vi "host-C-Experimental.vi"() -> (0 "K(Indicator)":fxp<+/-,64,32>=1.52587890625e-05, 1 "degree":dbl=0.1952712924057206, 2 "Nominal Freq":fxp<+/-,64,32>=0.494873046875)   [LabVIEW 2012]
uses:
  <vilib>/addons/control/pid/pid.llb/PID (DBL).vi
  <vilib>/Utility/file.llb/Write To Spreadsheet File (DBL).vi
  <vilib>/Utility/file.llb/Write To Spreadsheet File (I64).vi
  <vilib>/FPGAPlugInAG/PCI-7831R/niLvFpga_Open_PCI-7831R.vi
  <vilib>/rvi/interface/common/dynamic/niFpgaDynamicAddResources.vi
  <vilib>/Utility/error.llb/Error Cluster From Error Code.vi
  <vilib>/rvi/errors/niLvFpgaAdjustHostInterfaceError.vi
  <vilib>/FPGAPlugInAG/Dynamic/niLvFpga_Abort_Dynamic.vi
  <vilib>/FPGAPlugInAG/Dynamic/niLvFpga_Close_Dynamic.vi
  <vilib>/FPGAPlugInAG/PCI-7831R/niLvFpga_Abort_PCI-7831R.vi
  <vilib>/FPGAPlugInAG/PCI-7831R/niLvFpga_Close_PCI-7831R.vi
  <vilib>/FPGAPlugInAG/PCI-7831R/niLvFpga_Run_PCI-7831R.vi
  <vilib>/rvi/interface/nirviOpenFPGA/nirviOpenFPGA.xnode
  SB130-XPS/Documents/FPGA-project-apporach-retraction/FPGA Bitfiles/Apporach-Retract_FPGATarget_LIAFPGA3a-PDTest_MjY0boR9VLg.lvbitx
  Documents/Pramith_Computer/FPGA PLL/LIA_FPGA3a-PD Test-3.vi
  <vilib>/rvi/interface/nirviReadWriteControl/nirviReadWriteControl.xnode
  <vilib>/rvi/interface/nirviMethod/nirviMethod.xnode
  <vilib>/rvi/interface/nirviCloseFPGA/nirviCloseFPGA.xnode
  <vilib>/rvi/errors/niLvFpgaMergeErrorWithErrorCode.vi
  NiFpgaLv.dll
  <vilib>/FPGAPlugInAG/Dynamic/niLvFpga_StartFifo_Dynamic.vi
  <vilib>/FPGAPlugInAG/Dynamic/niLvFpga_StopFifo_Dynamic.vi
  <vilib>/rvi/interface/Simulation/niFpgaSimulationCallBeginRW.vi
  <vilib>/FPGAPlugInAG/Dynamic/niLvFpga_ReadFifo_Dynamic.vi
  <vilib>/addons/control/pid/NI_PID_pid.lvlib
panel:
  out "Output":dbl
  in  "Proportional Constant":dbl
  in  "Reinitialize":bool
  out "Numeric 2":dbl
  out "Corrected Frequency 2":dbl
  out "P+I Error 2":dbl
  in  "VCO Constant 2":dbl=0.010000000000000009
  out "Numeric 3":fxp<+/-,64,32>
  out "Sig Gen Frequency":dbl
  out "Corrected Frequency":fxp<+/-,64,32>
  out "Angular Frequency":fxp<+/-,64,32>
  out "Z Error":fxp<+/-,64,32>
  in  "VCO Constant":fxp<+/-,64,10>=0.010000000000000009
  in  "Proportional Gain":fxp<+/-,64,32>=0.0009999999310821295
  in  "Integral Gain":fxp<+/-,64,32>=0.0009999999310821295
  out "P+I Error":fxp<+/-,64,32>
  out "PID Input Error":dbl
  out "Phase (Degree) Shift":fxp<+/-,64,32>
  out "Numeric":fxp<+/-,64,32>
  out "For Proportional":fxp<+/-,64,32>
  out "Case Number":i16
  in  "Signal Generator":bool
  in  "PID":bool
  in  "Voltage (V)":dbl=0.03
  in  "Frequency":dbl=32767.0
  out "Waveform Chart 2":i32[](graph)
  out "Waveform Chart":i32[](graph)
  in  "Number of Elements":i32
  in  "Path 5":path
  in  "name-file 11":string="approach-15a"
  out "String 11":string
  in  "Path 7":path
  in  "name-file 9":string="approach-15a"
  out "String 9":string
  in  "Path 4":path
  in  "name-file 4":string="approach-15a"
  out "String 4":string
  in  "Path 3":path
  in  "name-file 3":string="approach-15a"
  out "String 3":string
  in  "Path 2":path
  in  "name-file 2":string="approach-15a"
  out "String 2":string
  in  "Data Collector":bool
  out "String":string
  in  "name-file":string="approach-15a"
  in  "Path":path
  out "Standardized nominal freq":dbl
  in  "Delta Nominal Frequency":dbl
  out "Ref":i32
  out "Sig":i32
  out "Sin":dbl(graph)
  out "Phase":dbl
  out "Ze Output":dbl=2.3841857910156248e-12
  out "The Decs":dbl=7.8125e-09
  out "LSB Weight":dbl=0.00030517578125
  in  "K":fxp<+,16,0>=6.103515625e-05
  in  "nominal freq 2":fxp<+,16,0>=0.494873046875
  out "x*y":dbl=0.015
  in  "stop 2":bool
  out "3rd stages":i32=1
  out "3rd decimation":i32=977
  out "1st decimation":i32=1
  out "2nd decimation":i32=128
  in  "Time Constant [s]":dbl=2.5 min=0.0 step=0.0001 format="%.2f"
  in  "Filter Rolloff":enum16{"20 dB", "40 dB", "60 dB", "80 dB"}(ring)
  out "Actual Sampling Frequency":dbl=200000.0
  in  "input range of 9205":dbl=10.0
  in  "Sampling Frequency":dbl=200000.0 min=1000.0 max=250000.0
  in  "stop":bool
  out "r":dbl(graph)=0.5098420210496609
  out "y":dbl=0.0017376029872894286
  out "x":dbl=0.5098390600609779
  out "f":dbl(graph)=31000.332441180944
  in  "dec2":i16=1
  in  "nominal freq":dbl=30000.0 min=500.0 max=125000.0
  in  "dec1":i16=1000
  in  "stages":i8=1 min=1 max=2
  in  "decimation":i16=1000
  # "Sampling Frequency"
  # "CIC First Decimation"
  # "MA Stages"
  # "CIC Second Decimation"
  # "PLL Nominal Frequency"
  # "MA Decimation"
  # "PLL Frequency Output"
  # "LIA Output"
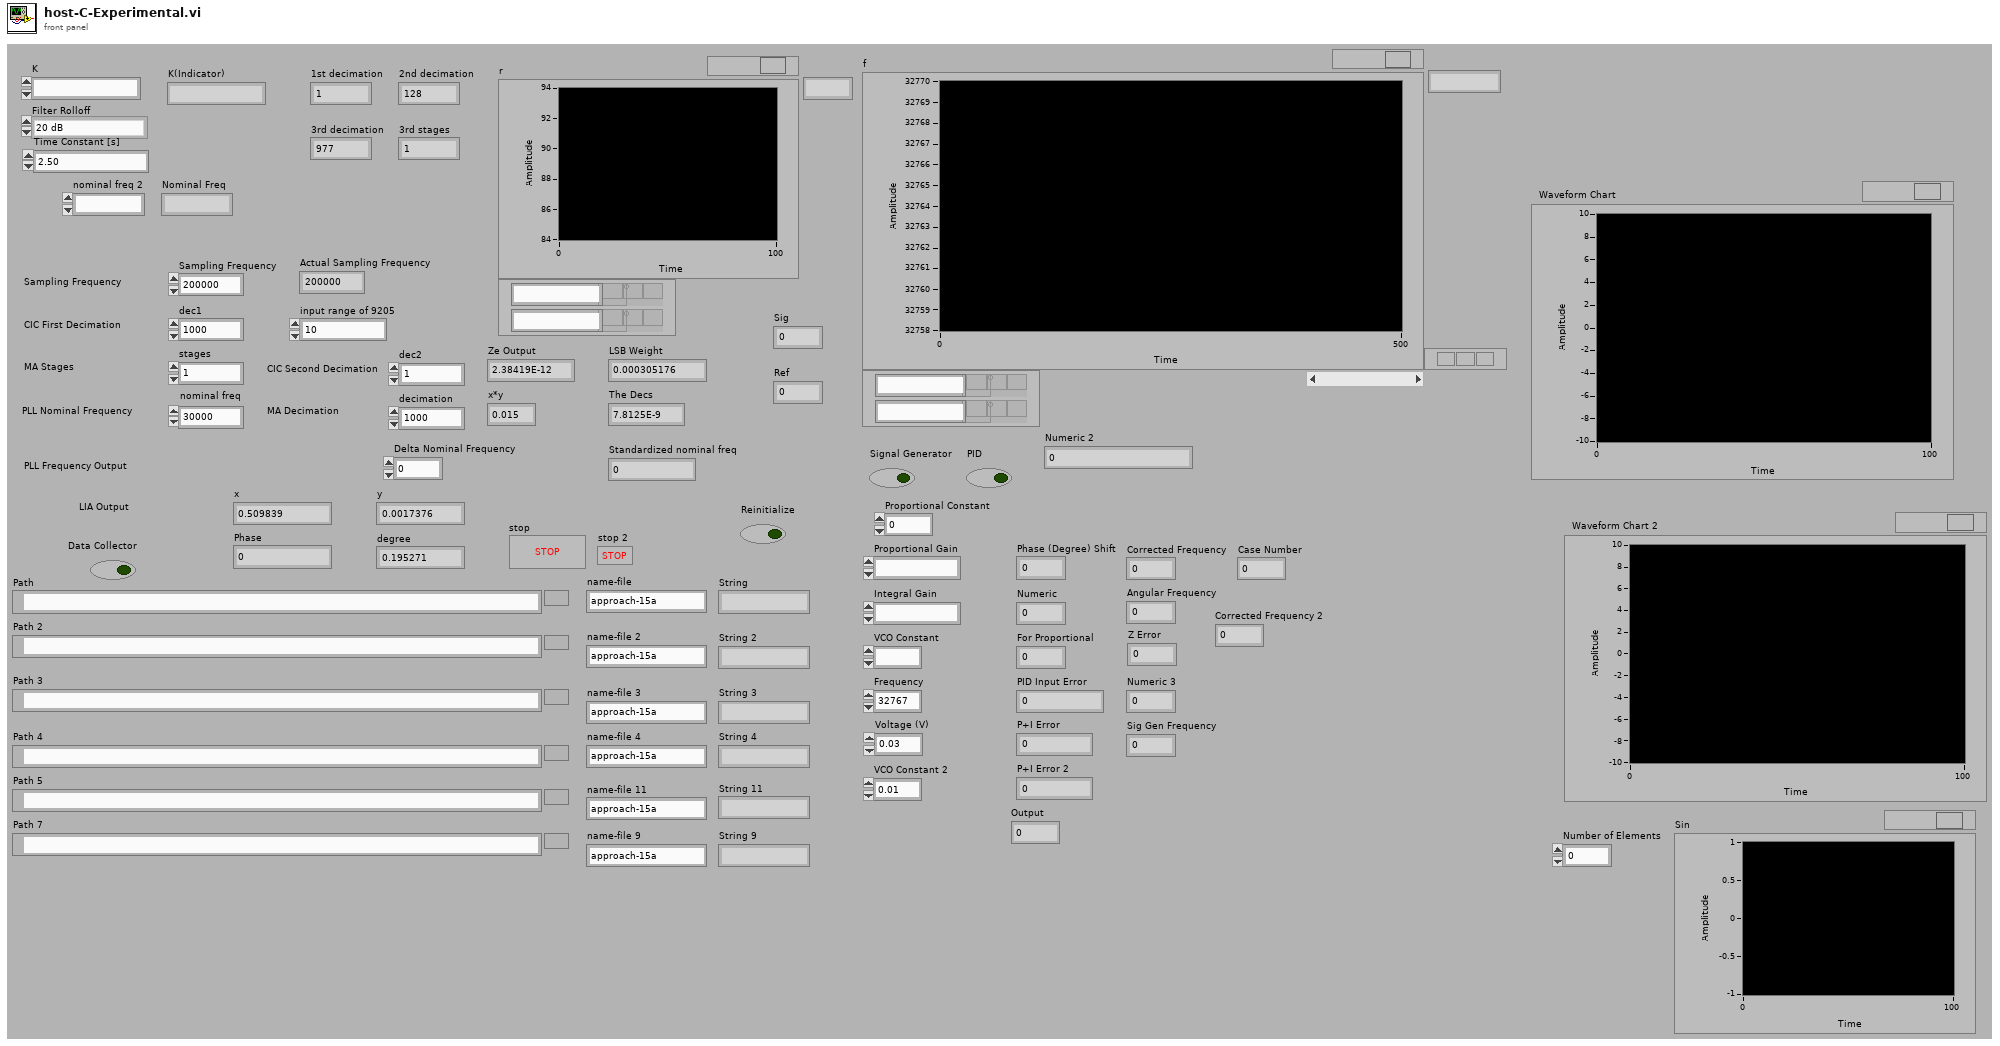
[diagram p1: front panel]
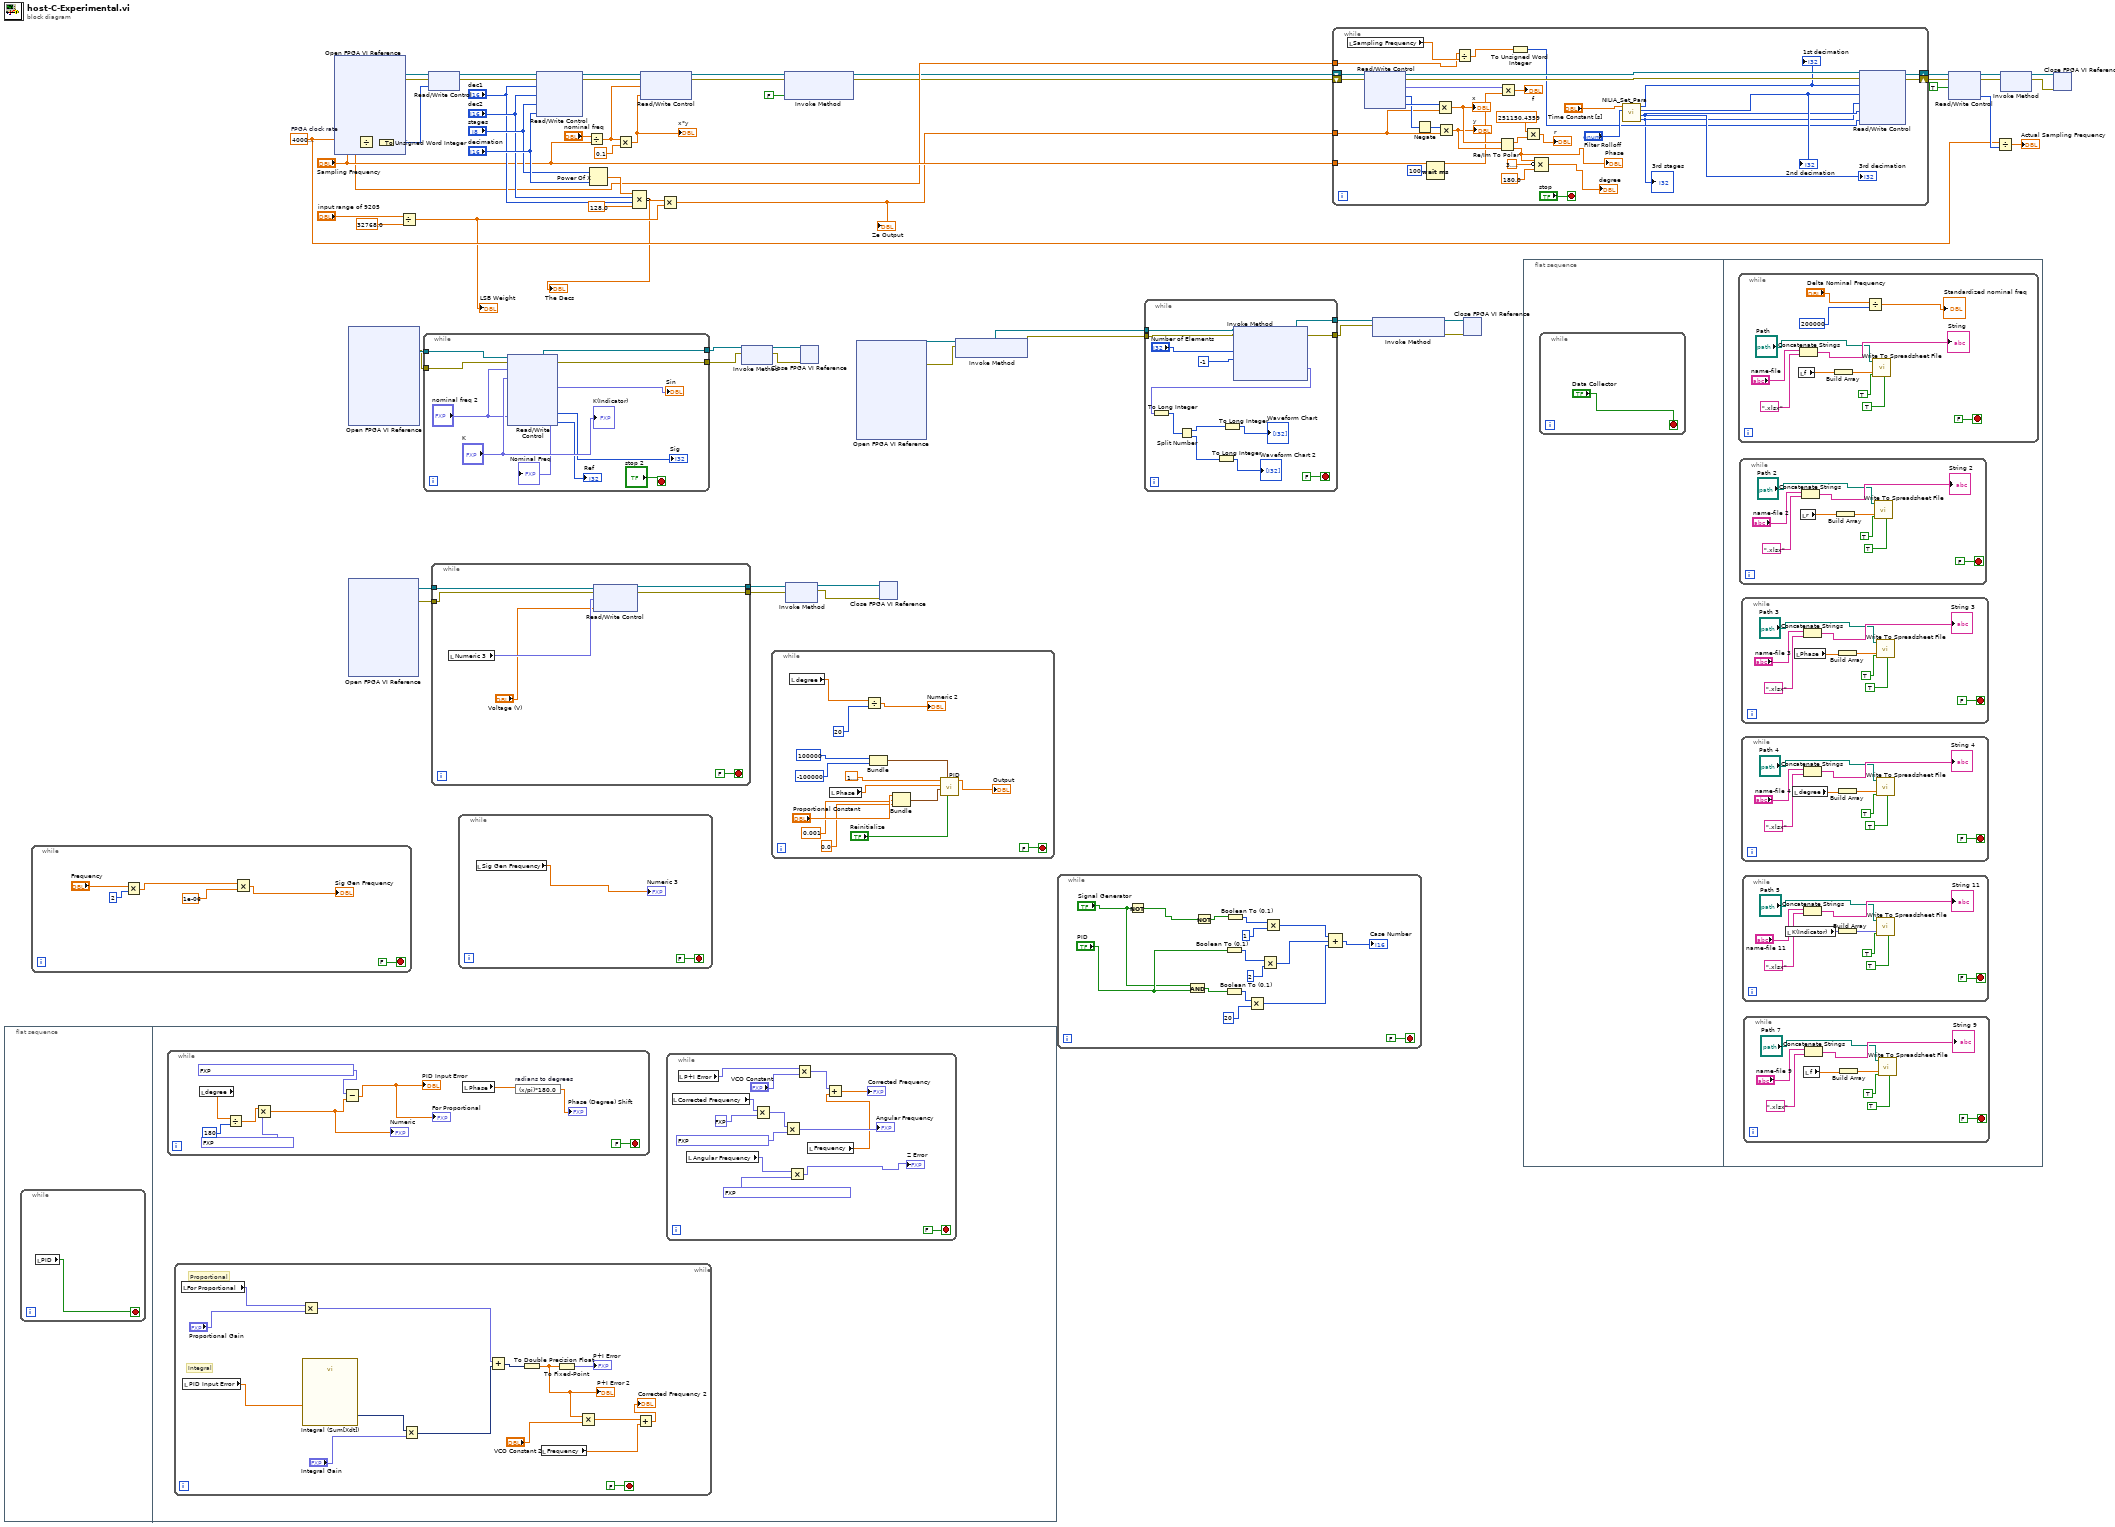
[diagram p0: block diagram]
diagram:
  w29 = 40000000.0  # FPGA clock rate
  n1 = flat-sequence {
    frame #0 {
      n2 = while {
        stop <- w60 stop-if-true
        n3 = local read "PID"() -> (w60:bool)
      }
    }
    frame #1 {
      n4 = while {
        stop <- FALSE stop-if-true
        n5 = local read "degree"() -> (w90:dbl)
        n6 = Divide(x=w90, y=i16 180) -> (x/y=w98:dbl)
        n7 = Multiply(x=w98, y=fxp<+,30,2> 3.1415926814079285) -> (x*y=w97:dbl)
        "Numeric" <- w97
        n8 = Subtract(x=fxp<+,50,1> 1.5707963199999995, y=w97) -> (x-y=→"PID Input Error" →"For Proportional":dbl)
        n9 = local read "Phase"() -> (w92:dbl)
        n10 = expression code="(x/pi)*180.0" "radians to degrees"(w92) -> (→"Phase (Degree) Shift":dbl)
      }
      n11 = while {
        stop <- FALSE stop-if-true
        # "Integral"
        # "Proportional"
        n12 = local read "For Proportional"() -> (w89:fxp<+/-,64,32>)
        n13 = local read "PID Input Error"() -> (w87:dbl)
        n14 = Multiply(x=w89, y="Proportional Gain") -> (x*y=w84:fxp<+/-,64,64>)
        n15 = call "Integral (Sum[Xdt])"("Signals"=w87) -> ("Result"=w86:dynamicdata)  [unwired: 5 in, 1 out]
        n16 = Multiply(x=w86, y="Integral Gain") -> (x*y=w83:dynamicdata)
        n17 = Add(x=w84, y=w83) -> (x+y=w82:dynamicdata)
        n18 = To Double Precision Float(number=w82) -> (double precision float=w79:dbl)
        "P+I Error 2" <- w79
        n19 = local read "Frequency"() -> (w76:dbl)
        n20 = To Fixed-Point(number=w79) -> (fixed-point=→"P+I Error":fxp<+/-,32,16>)  [unwired: 1 in]
        n21 = Multiply(x=w79, y="VCO Constant 2") -> (x*y=w77:dbl)
        n22 = Add(x=w77, y=w76) -> (x+y=→"Corrected Frequency 2":dbl)
      }
      n23 = while {
        stop <- FALSE stop-if-true
        n24 = local read "Corrected Frequency"() -> (w67:fxp<+/-,64,32>)
        n25 = local read "P+I Error"() -> (w63:fxp<+/-,64,32>)
        n26 = local read "Angular Frequency"() -> (w72:fxp<+/-,64,32>)
        n27 = Multiply(x=w67, y=fxp<+,1,2> 2.0) -> (x*y=w70:fxp<+/-,64,33>)
        n28 = Multiply(x=w70, y=fxp<+,30,2> 3.1415926814079285) -> (x*y=→"Angular Frequency":fxp<+/-,64,35>)
        n29 = Multiply(x=w72, y=fxp<+,46,7> 1.0000003385357559e-06) -> (x*y=→"Z Error":fxp<+/-,64,39>)
        n30 = Multiply(x=w63, y="VCO Constant") -> (x*y=w65:fxp<+/-,64,42>)
        n31 = local read "Frequency"() -> (w62:dbl)
        n32 = Add(x=w65, y=w62) -> (x+y=→"Corrected Frequency":dbl)
      }
    }
  }
  n33 = while {
    stop <- FALSE stop-if-true
    n34 = Multiply(x="Frequency", y=2) -> (x*y=w105:dbl)
    n35 = Multiply(x=w105, y=1e-06) -> (x*y=→"Sig Gen Frequency":dbl)
  }
  n36 = xnode "Open FPGA VI Reference"() -> ("FPGA VI Reference Out"=w35:refnum<k20>, "error out"=w34:errorcluster)  [unwired: 2 in]
  n37 = xnode ("Open FPGA VI Reference")() -> ("FPGA VI Reference Out"=w6:refnum<k20>, "error out"=w5:errorcluster)  [unwired: 2 in]
  n38 = xnode "Open FPGA VI Reference"() -> ("FPGA VI Reference Out"=w28:refnum<k20>, "error out"=w27:errorcluster)  [unwired: 2 in]
  n39 = Divide(x=w29, y="Sampling Frequency") -> (x/y=w41:dbl)
  n40 = To Unsigned Word Integer(number=w41) -> (unsigned 16bit integer=w40:u16)
  n41 = Divide(x="input range of 9205", y=32768.0) -> (x/y=w21:dbl)
  "LSB Weight" <- w21
  n42 = while {
    tunnel: w28 -> [w114]
    tunnel: w27 -> [w113]
    tunnel: [w112] -> w26
    tunnel: [w111] -> w25
    stop <- "stop 2" stop-if-true
    n43 = xnode "Read/Write Control"("FPGA VI Reference In"=w114, "error in"=w113, "nominal freq"="nominal freq 2", "K"="K") -> ("FPGA VI Reference Out"=w112:refnum<k20>, "error out"=w111:errorcluster, "Sin"=→"Sin":fxp<+/-,14,2>, "sig"=→"Sig":i16, "ref"=→"Ref":i16)  [unwired: 2 out]
    "K(Indicator)" <- "K"
    "Nominal Freq" <- "nominal freq 2"
  }
  n44 = xnode "Read/Write Control"("FPGA VI Reference In"=w35, "error in"=w34, "Period"=w40) -> ("FPGA VI Reference Out"=w43:refnum<k20>, "error out"=w42:errorcluster)
  n45 = while {
    tunnel: w6 -> [w121]
    tunnel: w5 -> [w120]
    tunnel: [w119] -> w4
    tunnel: [w118] -> w3
    stop <- FALSE stop-if-true
    n46 = local read "Numeric 3"() -> (w117:fxp<+/-,64,32>)
    n47 = xnode "Read/Write Control"("FPGA VI Reference In"=w121, "error in"=w120, "Z"=w117, "Voltage (V)"="Voltage (V)") -> ("FPGA VI Reference Out"=w119:refnum<k20>, "error out"=w118:errorcluster)
  }
  n48 = while {
    stop <- FALSE stop-if-true
    n49 = local read "Sig Gen Frequency"() -> (→"Numeric 3":dbl)
  }
  n50 = xnode "Read/Write Control"("FPGA VI Reference In"=w43, "error in"=w42, "dec1"="dec1", "dec2"="dec2", "stages"="stages", "decimation"="decimation") -> ("FPGA VI Reference Out"=w59:refnum<k20>, "error out"=w58:errorcluster)
  n51 = Divide(x="nominal freq", y="Sampling Frequency") -> (x/y=w37:dbl)
  n52 = Power Of X(1:"decimation", 2:"stages") -> (0:w54:dbl)
  n53 = Multiply(x=w37, y=0.1) -> (x*y=w22:dbl)
  "x*y" <- w22
  n54 = Compound Arithmetic op=MULTIPLY(w54, "dec2", "dec1", 128.0) -> (invert w20:dbl)
  "The Decs" <- w20
  n55 = xnode "Read/Write Control"("FPGA VI Reference In"=w59, "error in"=w58, "nominal freq"=w37, "K"=w22) -> ("FPGA VI Reference Out"=w10:refnum<k20>, "error out"=w9:errorcluster)
  n56 = Multiply(x=w20, y=w21) -> (x*y=w19:dbl)
  "Ze Output" <- w19
  n57 = xnode "Invoke Method"("FPGA VI Reference In"=w26, "error in"=w25) -> ("FPGA VI Reference Out"=w24:refnum<k20>, "error out"=w23:errorcluster)
  n58 = while {
    stop <- FALSE stop-if-true
    n59 = local read "degree"() -> (w133:dbl)
    n60 = local read "Phase"() -> (w132:dbl)
    n61 = Divide(x=w133, y=20) -> (x/y=→"Numeric 2":dbl)
    n62 = Bundle(100000, -100000) -> (w136:cluster{i32, i32})  [unwired: 1 in]
    n63 = Bundle("Proportional Constant"="Proportional Constant", 0.001, 0.0) -> (w129:cluster{"Proportional Constant":dbl, dbl, dbl})  [unwired: 1 in]
    n64 = call-poly <vilib>:"PID.vi"("reinitialize? (F)"="Reinitialize", "output range"=w136, "PID gains"=w129, "process variable"=w132, "setpoint"=1.5707963267948966) -> ("output"=→"Output":dbl)  [unwired: 5 in, 1 out]
  }
  n65 = xnode "Invoke Method"("FPGA VI Reference In"=w10, "error in"=w9, "Wait Until Done (F)"=FALSE) -> ("FPGA VI Reference Out"=w8:refnum<k20>, "error out"=w7:errorcluster)
  n66 = xnode "Invoke Method"("FPGA VI Reference In"=w4, "error in"=w3) -> ("FPGA VI Reference Out"=w2:refnum<k20>, "error out"=w1:errorcluster)
  n67 = xnode "Close FPGA VI Reference"("FPGA VI Reference In"=w24, "error in"=w23) -> ()  [unwired: 1 out]
  n68 = xnode "Open FPGA VI Reference"() -> ("FPGA VI Reference Out"=w18:refnum<k20>, "error out"=w17:errorcluster)  [unwired: 2 in]
  n69 = xnode "Close FPGA VI Reference"("FPGA VI Reference In"=w2, "error in"=w1) -> ()  [unwired: 1 out]
  n70 = xnode "Invoke Method"("FPGA VI Reference In"=w18, "error in"=w17) -> ("FPGA VI Reference Out"=w16:refnum<k20>, "error out"=w15:errorcluster)
  n71 = while {
    stop <- FALSE stop-if-true
    n72 = Not(x="Signal Generator") -> (.not. x?=w142:bool)
    n73 = And(x="Signal Generator", y="PID") -> (x .and. y?=w154:bool)
    n74 = Not(x=w142) -> (.not. x?=w141:bool)
    n75 = Boolean To (0,1)(Boolean="PID") -> (0, 1=w146:i16)
    n76 = Boolean To (0,1)(Boolean=w154) -> (0, 1=w153:i16)
    n77 = Boolean To (0,1)(Boolean=w141) -> (0, 1=w147:i16)
    n78 = Multiply(x=w153, y=20) -> (x*y=w151:i32)
    n79 = Multiply(x=w146, y=2) -> (x*y=w143:i32)
    n80 = Multiply(x=w147, y=1) -> (x*y=w144:i32)
    n81 = Compound Arithmetic op=ADD(w144, w143, w151) -> (→"Case Number":i32)
  }
  n82 = while {
    tunnel: w16 -> [w163]
    tunnel: w15 -> [w162]
    tunnel: [w161] -> w12
    tunnel: [w160] -> w11
    stop <- FALSE stop-if-true
    n83 = xnode "Invoke Method"("FPGA VI Reference In"=w163, "error in"=w162, "Number of Elements"="Number of Elements", "Timeout (ms)"=-1) -> ("FPGA VI Reference Out"=w161:refnum<k20>, "error out"=w160:errorcluster, "Data"=w156:fxp<+/-,64,16>[])  [unwired: 1 out]
    n84 = To Long Integer(number=w156) -> (32bit integer=w157:i32[])
    n85 = Split Number(x=w157) -> (hi(x)=w167:u16[], lo(x)=w166:u16[])
    n86 = To Long Integer(number=w166) -> (32bit integer=→"Waveform Chart 2":i32[])
    n87 = To Long Integer(number=w167) -> (32bit integer=→"Waveform Chart":i32[])
  }
  n88 = while {
    shift-right: [w185] -> w50
    shift-left: w8 -> [w200]
    shift-right: [w184] -> w49
    shift-left: w7 -> [w199]
    tunnel: w19 -> [w196]
    tunnel: "Sampling Frequency" -> [w188]
    tunnel: w29 -> [w177]
    stop <- "stop" stop-if-true
    n89 = local read "Sampling Frequency"() -> (w178:dbl)
    n90 = xnode "Read/Write Control"("FPGA VI Reference In"=w200, "error in"=w199) -> ("FPGA VI Reference Out"=w185:refnum<k20>, "error out"=w184:errorcluster, "f"=w189:fxp<+/-,32,0>, "channelQ"=w197:i64, "channelI"=w198:i64)
    n91 = Negate(x=w197) -> (-x=w186:i64)
    n92 = Wait (ms)(milliseconds to wait=u32 100) -> ()  [unwired: 1 out]
    n93 = Multiply(x=w198, y=w196) -> (x*y=w195:dbl)
    "x" <- w195
    n94 = Multiply(x=w186, y=w196) -> (x*y=w194:dbl)
    "y" <- w194
    n95 = Divide(x=w177, y=w178) -> (x/y=w176:dbl)
    n96 = Re/Im To Polar(2:w194, 3:w195) -> (0:w169:dbl, 1:w172:dbl)
    "Phase" <- w169
    n97 = Multiply(x=w189, y=w188) -> (x*y=→"f":dbl)
    n98 = To Unsigned Word Integer(number=w176) -> (unsigned 16bit integer=w175:u16)
    n99 = Multiply(x=251150.4359, y=w172) -> (x*y=→"r":dbl)
    n100 = Compound Arithmetic op=MULTIPLY(w169, invert 3.141592653589793, 180.0 ("value")) -> (→"degree":dbl)
    n101 = call "NILIA_Set_Para.vi"("rolloff"="Filter Rolloff", "TC [sec]"="Time Constant [s]") -> ("3rd stages"=w174:i32, "3rd decimation"=w179:i32, "2nd decimation"=w180:i32, "1st decimation"=w181:i32)  [unwired: 5 in, 1 out]
    "2nd decimation" <- w180
    "1st decimation" <- w181
    "3rd decimation" <- w179
    "3rd stages" <- w174
    n102 = xnode "Read/Write Control"("FPGA VI Reference In"=w185, "error in"=w184, "dec1"=w181, "dec2"=w180, "stages"=w174, "decimation"=w179, "Period"=w175) -> ()  [unwired: 2 out]
  }
  n103 = xnode "Invoke Method"("FPGA VI Reference In"=w12, "error in"=w11) -> ("FPGA VI Reference Out"=w14:refnum<k20>, "error out"=w13:errorcluster)
  n104 = xnode "Close FPGA VI Reference"("FPGA VI Reference In"=w14, "error in"=w13) -> ()  [unwired: 1 out]
  n105 = flat-sequence {
    frame #0 {
      n106 = while {
        stop <- "Data Collector" stop-if-true
      }
    }
    frame #1 {
      n107 = while {
        stop <- FALSE stop-if-true
        n108 = local read "f"() -> (w254:dbl)
        n109 = Concatenate Strings("name-file", ".xlsx") -> (→"String":string)
        n110 = Build Array(w254) -> (w253:dbl[])
        n111 = Divide(x="Delta Nominal Frequency", y=200000) -> (x/y=→"Standardized nominal freq":dbl)
        n112 = call-poly <vilib>:"Write To Spreadsheet File.vi"("transpose? (no:F)"=TRUE, "append to file? (new file:F)"=TRUE, "1D data"=w253, "file path (dialog if empty)"="Path") -> ()  [unwired: 4 in, 1 out]
      }
      n113 = while {
        stop <- FALSE stop-if-true
        n114 = local read "r"() -> (w245:dbl)
        n115 = Concatenate Strings("name-file 2", ".xlsx") -> (→"String 2":string)
        n116 = Build Array(w245) -> (w244:dbl[])
        n117 = call-poly <vilib>:"Write To Spreadsheet File.vi"("transpose? (no:F)"=TRUE, "append to file? (new file:F)"=TRUE, "1D data"=w244, "file path (dialog if empty)"="Path 2") -> ()  [unwired: 4 in, 1 out]
      }
      n118 = while {
        stop <- FALSE stop-if-true
        n119 = local read "Phase"() -> (w236:dbl)
        n120 = Concatenate Strings("name-file 3", ".xlsx") -> (→"String 3":string)
        n121 = Build Array(w236) -> (w235:dbl[])
        n122 = call-poly <vilib>:"Write To Spreadsheet File.vi"("transpose? (no:F)"=TRUE, "append to file? (new file:F)"=TRUE, "1D data"=w235, "file path (dialog if empty)"="Path 3") -> ()  [unwired: 4 in, 1 out]
      }
      n123 = while {
        stop <- FALSE stop-if-true
        n124 = local read "degree"() -> (w227:dbl)
        n125 = Concatenate Strings("name-file 4", ".xlsx") -> (→"String 4":string)
        n126 = Build Array(w227) -> (w226:dbl[])
        n127 = call-poly <vilib>:"Write To Spreadsheet File.vi"("transpose? (no:F)"=TRUE, "append to file? (new file:F)"=TRUE, "1D data"=w226, "file path (dialog if empty)"="Path 4") -> ()  [unwired: 4 in, 1 out]
      }
      n128 = while {
        stop <- FALSE stop-if-true
        n129 = local read "K(Indicator)"() -> (w209:fxp<+/-,64,32>)
        n130 = Concatenate Strings("name-file 11", ".xlsx") -> (→"String 11":string)
        n131 = Build Array(w209) -> (w208:fxp<+/-,64,32>[])
        n132 = call-poly <vilib>:"Write To Spreadsheet File.vi"("transpose? (no:F)"=TRUE, "append to file? (new file:F)"=TRUE, "1D data"=w208, "file path (dialog if empty)"="Path 5") -> ()  [unwired: 4 in, 1 out]
      }
      n133 = while {
        stop <- FALSE stop-if-true
        n134 = local read "f"() -> (w218:dbl)
        n135 = Concatenate Strings("name-file 9", ".xlsx") -> (→"String 9":string)
        n136 = Build Array(w218) -> (w217:dbl[])
        n137 = call-poly <vilib>:"Write To Spreadsheet File.vi"("transpose? (no:F)"=TRUE, "append to file? (new file:F)"=TRUE, "1D data"=w217, "file path (dialog if empty)"="Path 7") -> ()  [unwired: 4 in, 1 out]
      }
    }
  }
  n138 = xnode "Read/Write Control"("FPGA VI Reference In"=w50, "error in"=w49, "stop"=TRUE) -> ("FPGA VI Reference Out"=w47:refnum<k20>, "error out"=w46:errorcluster, "ticks"=w31:u16)
  n139 = Divide(x=w29, y=w31) -> (x/y=→"Actual Sampling Frequency":dbl)
  n140 = xnode "Invoke Method"("FPGA VI Reference In"=w47, "error in"=w46) -> ("FPGA VI Reference Out"=w45:refnum<k20>, "error out"=w44:errorcluster)
  n141 = xnode "Close FPGA VI Reference"("FPGA VI Reference In"=w45, "error in"=w44) -> ()  [unwired: 1 out]
